vi "Pre Launch Init.vi"(11 "Panel Actor in":refnum<class "Panel Actor.lvclass">) -> (0 "error out":errorcluster, 3 "Panel Actor out":refnum<class "Panel Actor.lvclass">)   [LabVIEW 2017, in "MGI-Panel Actor.lvlib" / "Panel Actor.lvclass"]
doc: "Initializes the panel actor. Creates the Panel Helper.\n\n----\nCopyright: MGI 2018\nAuthor: Derek Trepanier"
uses:
  Panel Actor.lvclass
  panel-manager/Source/Panel Helper/Panel Helper.lvclass
  <vilib>/ActorFramework/Actor/Actor.lvclass
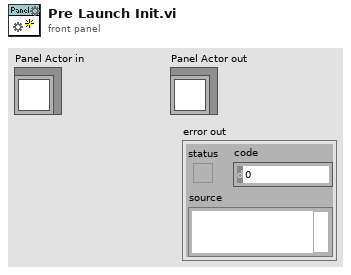
[diagram p1: front panel]
types:
  T1 = typedef "MGI-Panel Manager.lvlib/Panel Helper.lvclass/Panel Events.ctl" = cluster{"My Panel":refnum<user-event>, "Top Level Initialized":refnum<user-event>}
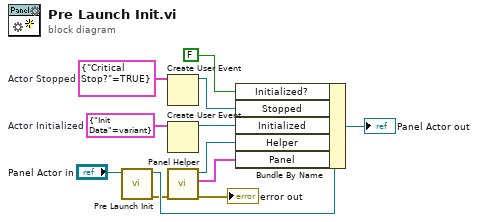
[diagram p0: block diagram]
diagram:
  w5 = cluster{"Init Data":variant} {"Init Data"=variant}  # Actor Initialized
  w10 = cluster{"Critical Stop?":bool} {"Critical Stop?"=TRUE}  # Actor Stopped
  n1 = call-parent "Pre Launch Init.vi"("Actor in"="Panel Actor in") -> ("error out"=w2:errorcluster, "Actor out"=w11:refnum<class "Panel Actor.lvclass">)  [unwired: 9 in]
  n2 = Create User Event(user event datatype=w10) -> (user event=w9:refnum<user-event>)  [unwired: 1 in, 1 out]
  n3 = Create User Event(user event datatype=w5) -> (user event=w3:refnum<user-event>)  [unwired: 1 in, 1 out]
  n4 = call "Panel Helper.vi"("Error In"=w2) -> ("Error Out"=→"error out":errorcluster, "Panel Events"=w1:T1, "Panel Helper out"=w6:refnum<class "Panel Helper.lvclass">)  [unwired: 8 in]
  n5 = Bundle By Name(cluster=w11, "Initialized?"=FALSE, "Stopped"=w9, "Initialized"=w3, "Helper"=w6, "Panel"=w1) -> (→"Panel Actor out":refnum<class "Panel Actor.lvclass">)
